vi "LV_VIDEO_3_PROJECT_2.vi"() -> ()   [LabVIEW 2022 SP3]
panel:
  out "Minutes":dbl
  out "Message":string
  out "Warning":bool
  out "Seconds":dbl
  out "Hours":dbl
  in  "Total Time in Seconds":dbl
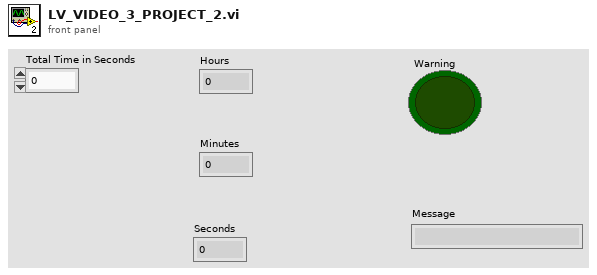
[diagram p1: front panel]
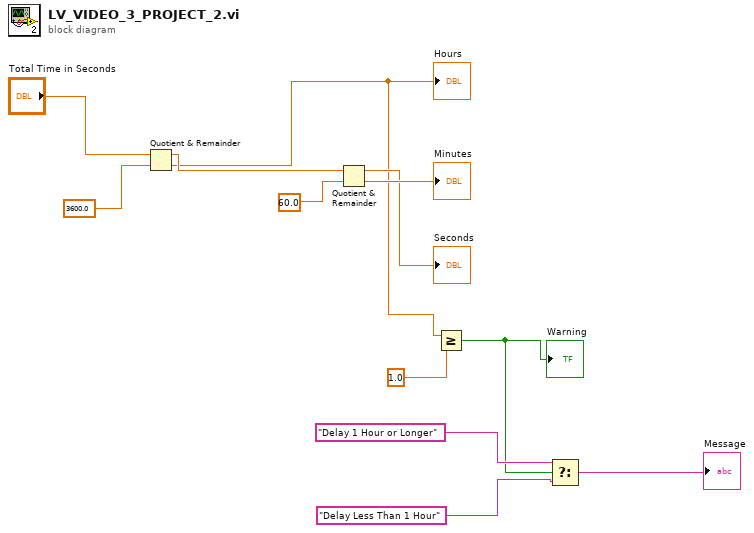
[diagram p0: block diagram]
diagram:
  n1 = Quotient & Remainder(x="Total Time in Seconds", y=3600.0 ("x")) -> (x-y*floor(x/y)=w10:dbl, floor(x/y)=w6:dbl)
  "Hours" <- w6
  n2 = Quotient & Remainder(x=w10, y=60.0 ("x-y*floor(x/y)")) -> (x-y*floor(x/y)=→"Seconds":dbl, floor(x/y)=→"Minutes":dbl)
  n3 = Greater Or Equal?(x=w6, y=1.0) -> (x >= y?=w3:bool)
  "Warning" <- w3
  n4 = Select(t="Delay 1 Hour or Longer", s=w3, f="Delay Less Than 1 Hour") -> (s? t:f=→"Message":string)
